vi "m1m3_putSample_InclinometerData.vi"(8 "error in (no error)":errorcluster, 11 "InclinometerData_Ctl":T1) -> (0 "error out":errorcluster, 2 "function return":i32, 3 "InclinometerData_Ctl out":T1)   [LabVIEW 2016, in "SALLV_m1m3.lvlib"]
doc: "int m1m3_shm_putSample_InclinometerDataLV(m1m3_InclinometerDataLV *InclinometerData_Ctl );"
uses:
  SALLV_m1m3.lvlib
  DataTypes/InclinometerData.ctl
  SALLV_m1m3.so
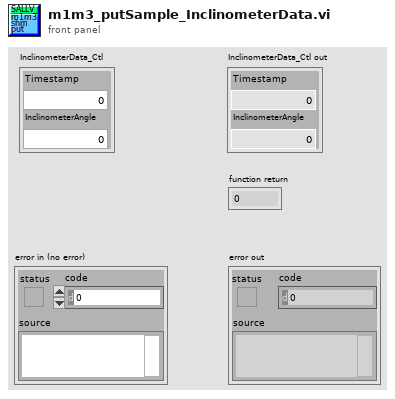
[diagram p1: front panel]
types:
  T1 = typedef "SALLV_m1m3.lvlib/InclinometerData.ctl" = cluster{"Timestamp":dbl, "InclinometerAngle":sgl}
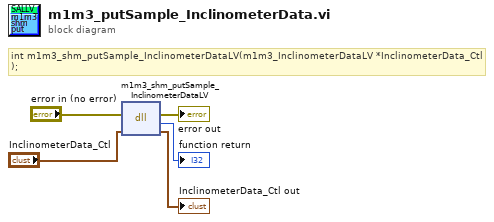
[diagram p0: block diagram]
diagram:
  # "int m1m3_shm_putSample_InclinometerDataLV(m1m3_InclinometerDataLV *InclinometerData_Ctl );"
  n1 = dll-call lib="opt/CODE/SALLV_m1m3/SALLV_m1m3.*" fn="m1m3_shm_putSample_InclinometerDataLV"(error in="error in (no error)", "InclinometerData_Ctl"="InclinometerData_Ctl") -> (error out=→"error out":errorcluster, →"function return":i32, "InclinometerData_Ctl"=→"InclinometerData_Ctl out":T1)  [unwired: 2 in, 1 out]
